vi "Protocol.RQST Lookup Table.vi"(7 "Action":T3, 8 "error in (no error)":errorcluster, 9 "ID":u32, 10 "Data":T2, 11 "Rqst LUT":T1) -> (0 "error out":errorcluster, 1 "Found?":bool, 2 "Data Out":T2, 3 "Rqst LUT out":T1, 5 "# of Active Requests":i32)   [LabVIEW 2019, in "J1939 Addon Engine.lvlib"]
uses:
  J1939 Addon Engine.lvlib
  Types/Protocol.RQST Lookup Table Cluster.ctl
  <vilib>/xnet/xnet.llb/XNET Frame CAN.ctl
  <vilib>/xnet/xnet.llb/XNET Frame Type CAN.ctl
  Types/Protocol.RQST Lookup Table Action.ctl
  Types/Protocol.RQST Lookup Table Reference.ctl
panel:
  # "OUTPUTS"
  # "INPUTS"
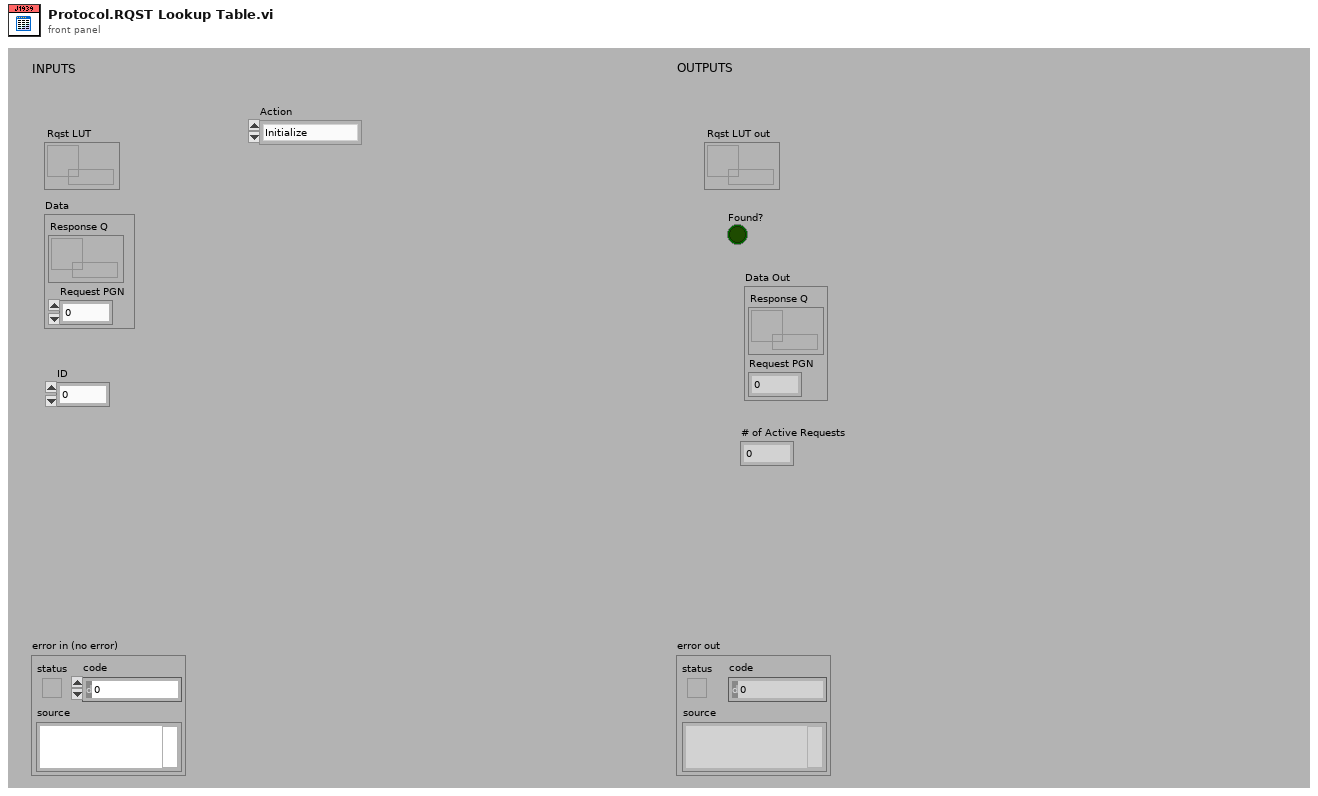
[diagram p1: front panel]
types:
  T1 = typedef "J1939 Addon Engine.lvlib/Protocol.RQST Lookup Table Reference.ctl" = refnum<data-value>
  T2 = typedef "J1939 Addon Engine.lvlib/Protocol.RQST Lookup Table Cluster.ctl" = cluster{"Response Q":refnum<queue>, "Request PGN":u32}
  T3 = typedef "J1939 Addon Engine.lvlib/Protocol.RQST Lookup Table Action.ctl" = enum16{"Initialize", "Add", "Get", "Remove", "Get Active Requests"}
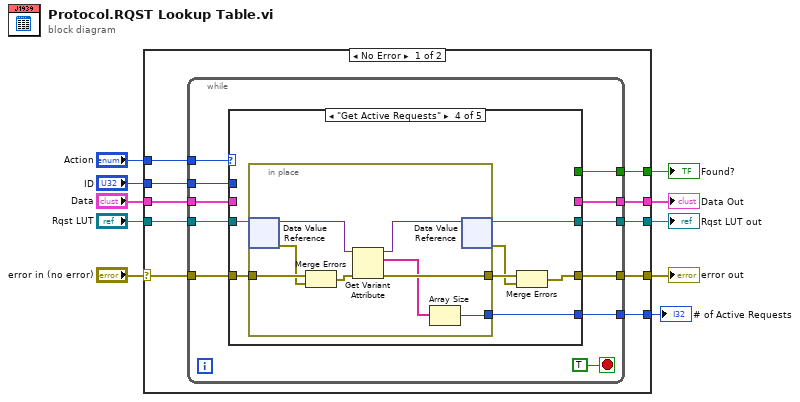
[diagram p0: block diagram]
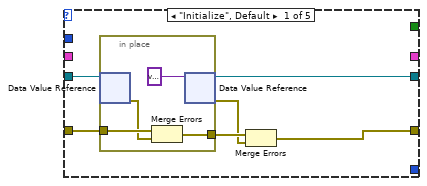
[diagram p2: hidden frame]
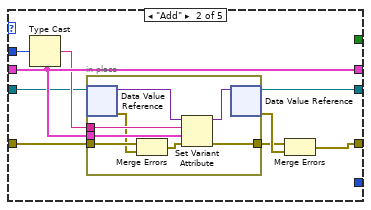
[diagram p3: hidden frame]
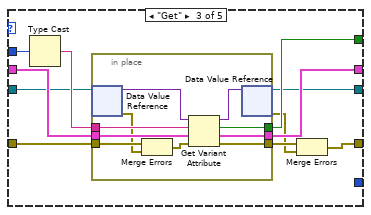
[diagram p4: hidden frame]
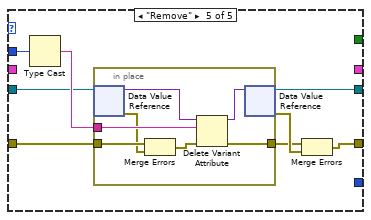
[diagram p5: hidden frame]
diagram:
  n1 = case shown="No Error" "error in (no error)" {
    selector: "error in (no error)" -> [w16 w111]
    tunnel: [w15 w111] -> w9
    tunnel: "Data" -> [w19 _]
    tunnel: "Action" -> [w20 _]
    tunnel: [w18 _] -> w6
    tunnel: "ID" -> [w17 _]
    tunnel: [w14 _] -> w4
    tunnel: "Rqst LUT" -> [w13 w110]
    tunnel: [w12 w110] -> w2
    tunnel: [w11 _] -> w1
    frame No Error {
      n2 = while {
        tunnel: w20 -> [w31]
        tunnel: w19 -> [w30]
        tunnel: [w28] -> w18
        tunnel: w17 -> [w27]
        tunnel: w16 -> [w26]
        tunnel: [w25] -> w15
        tunnel: [w24] -> w14
        tunnel: w13 -> [w23]
        tunnel: [w22] -> w12
        tunnel: [w21] -> w11
        stop <- TRUE stop-if-true
        n3 = case shown="\"Get Active Requests\"" w31 {
          tunnel: w30 -> [_ w50 w65 _ _]
          tunnel: [_ w50 w64 _ _] -> w28
          tunnel: w27 -> [_ w49 w69 _ w102]
          tunnel: w26 -> [w35 w47 w67 w86 w101]
          tunnel: [w32 w43 w61 w83 w96] -> w25
          tunnel: [_ _ w63 _ _] -> w24
          tunnel: w23 -> [w37 w46 w62 w84 w99]
          tunnel: [w36 w45 w59 w81 w98] -> w22
          tunnel: [_ _ _ w80 _] -> w21
          frame "Initialize", Default {
            n4 = in-place {
              in-place-border: w35 -> [w40]
              in-place-border: [w38] -> w34
              n5 = in-place-dvr #1(w37) -> (w39:errorcluster)  [unwired: 1 out]
              n6 = Merge Errors(w40, w39) -> (w38:errorcluster)
              n7 = in-place-dvr #1(variant ("duplicate variant")) -> (w36:T1, w33:errorcluster)
            }
            n8 = Merge Errors(w34, w33) -> (w32:errorcluster)
          }
          frame "Add" {
            n9 = Type Cast(x=w49) -> (*(type *) &x=w48:string)  [unwired: 1 in]
            n10 = in-place {
              in-place-border: w50 -> [w58]
              in-place-border: w48 -> [w57]
              in-place-border: w47 -> [w56]
              in-place-border: [w55] -> w42
              n11 = in-place-dvr #2(w46) -> (w54:variant, w51:errorcluster)
              n12 = Merge Errors(w56, w51) -> (w52:errorcluster)
              n13 = Set Variant Attribute(Variant=w54, name=w57, value=w58, error in=w52) -> (Variant out=w53:variant, error out=w55:errorcluster)  [unwired: 1 out]
              n14 = in-place-dvr #2(w53) -> (w45:T1, w44:errorcluster)
            }
            n15 = Merge Errors(w42, w44) -> (w43:errorcluster)
          }
          frame "Get" {
            n16 = Type Cast(x=w69) -> (*(type *) &x=w68:string)  [unwired: 1 in]
            n17 = in-place {
              in-place-border: w68 -> [w79]
              in-place-border: w67 -> [w78]
              in-place-border: [w77] -> w66
              in-place-border: w65 -> [w76]
              in-place-border: [w75] -> w64
              in-place-border: [w74] -> w63
              n18 = in-place-dvr #3(w62) -> (w73:variant, w70:errorcluster)
              n19 = Merge Errors(w78, w70) -> (w71:errorcluster)
              n20 = Get Variant Attribute(Variant=w73, name=w79, default value (empty Variant)=w76, error in=w71) -> (duplicate Variant=w72:variant, found=w74:bool, value=w75:T2, error out=w77:errorcluster)
              n21 = in-place-dvr #3(w72) -> (w59:T1, w60:errorcluster)
            }
            n22 = Merge Errors(w66, w60) -> (w61:errorcluster)
          }
          frame "Get Active Requests" {
            n23 = in-place {
              in-place-border: w86 -> [w94]
              in-place-border: [w93] -> w85
              in-place-border: [w87] -> w80
              n24 = in-place-dvr #4(w84) -> (w92:variant, w89:errorcluster)
              n25 = Merge Errors(w94, w89) -> (w90:errorcluster)
              n26 = Get Variant Attribute(Variant=w92, error in=w90) -> (duplicate Variant=w91:variant, names=w88:string[], error out=w93:errorcluster)  [unwired: 2 in, 1 out]
              n27 = Array Size(array=w88) -> (size(s)=w87:i32)
              n28 = in-place-dvr #4(w91) -> (w81:T1, w82:errorcluster)
            }
            n29 = Merge Errors(w85, w82) -> (w83:errorcluster)
          }
          frame "Remove" {
            n30 = Type Cast(x=w102) -> (*(type *) &x=w100:string)  [unwired: 1 in]
            n31 = in-place {
              in-place-border: w101 -> [w109]
              in-place-border: [w108] -> w95
              in-place-border: w100 -> [w107]
              n32 = in-place-dvr #5(w99) -> (w106:variant, w104:errorcluster)
              n33 = Merge Errors(w109, w104) -> (w105:errorcluster)
              n34 = Delete Variant Attribute(4:w105, 6:w107, 7:w106) -> (0:w108:errorcluster, 3:w103:variant)  [unwired: 1 out]
              n35 = in-place-dvr #5(w103) -> (w98:T1, w97:errorcluster)
            }
            n36 = Merge Errors(w95, w97) -> (w96:errorcluster)
          }
        }
      }
    }
    frame Error {
    }
  }
  "error out" <- w9
  "Data Out" <- w6
  "Found?" <- w4
  "Rqst LUT out" <- w2
  "# of Active Requests" <- w1
